vi "test_CCDSetAndGetGain.vi"(6 "Delay between send and receive [ms]":i32=100, 7 "Test should pass":bool=TRUE, 8 "error in":errorcluster, 9 "tear down connection":bool=TRUE, 10 "set-up a connection":bool=TRUE, 11 "device selection":enum16{"monochromator", "CCD", "SCD"}(ring)=enum."CCD") -> (0 "error out":errorcluster)   [LabVIEW 2023]
uses:
  Classes/CCD/GainTokenEnum.ctl
  Classes/CCD/CCD.lvclass
  <vilib>/addons/_JKI Toolkits/Caraya/classes/Assert/Assert Equal Value and Type_Variant.vi
  <vilib>/addons/_JKI Toolkits/Caraya/classes/Assert/Assert Not Error.vi
  <vilib>/addons/_JKI Toolkits/Caraya/classes/Test/Test.lvclass
  <vilib>/addons/_JKI Toolkits/Caraya/classes/Assert/Assert.lvclass
panel:
  # "Connector Pane"
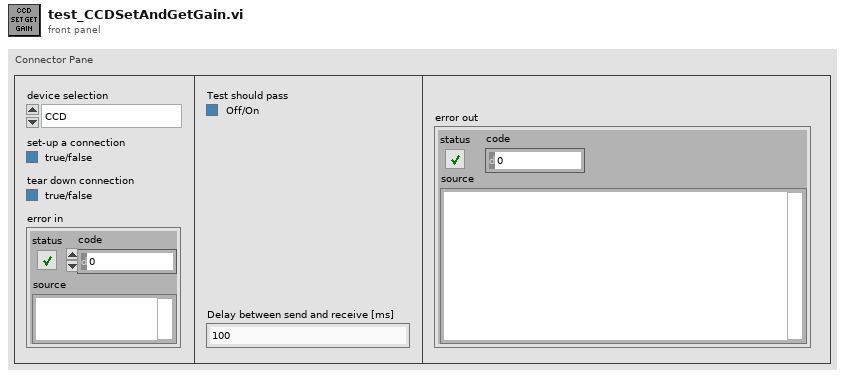
[diagram p1: front panel]
types:
  T1 = typedef "CCD.lvclass/GainTokenEnum.ctl" = enum16{"High Light", "Best Dynamic Range", "High Sensitivity"}
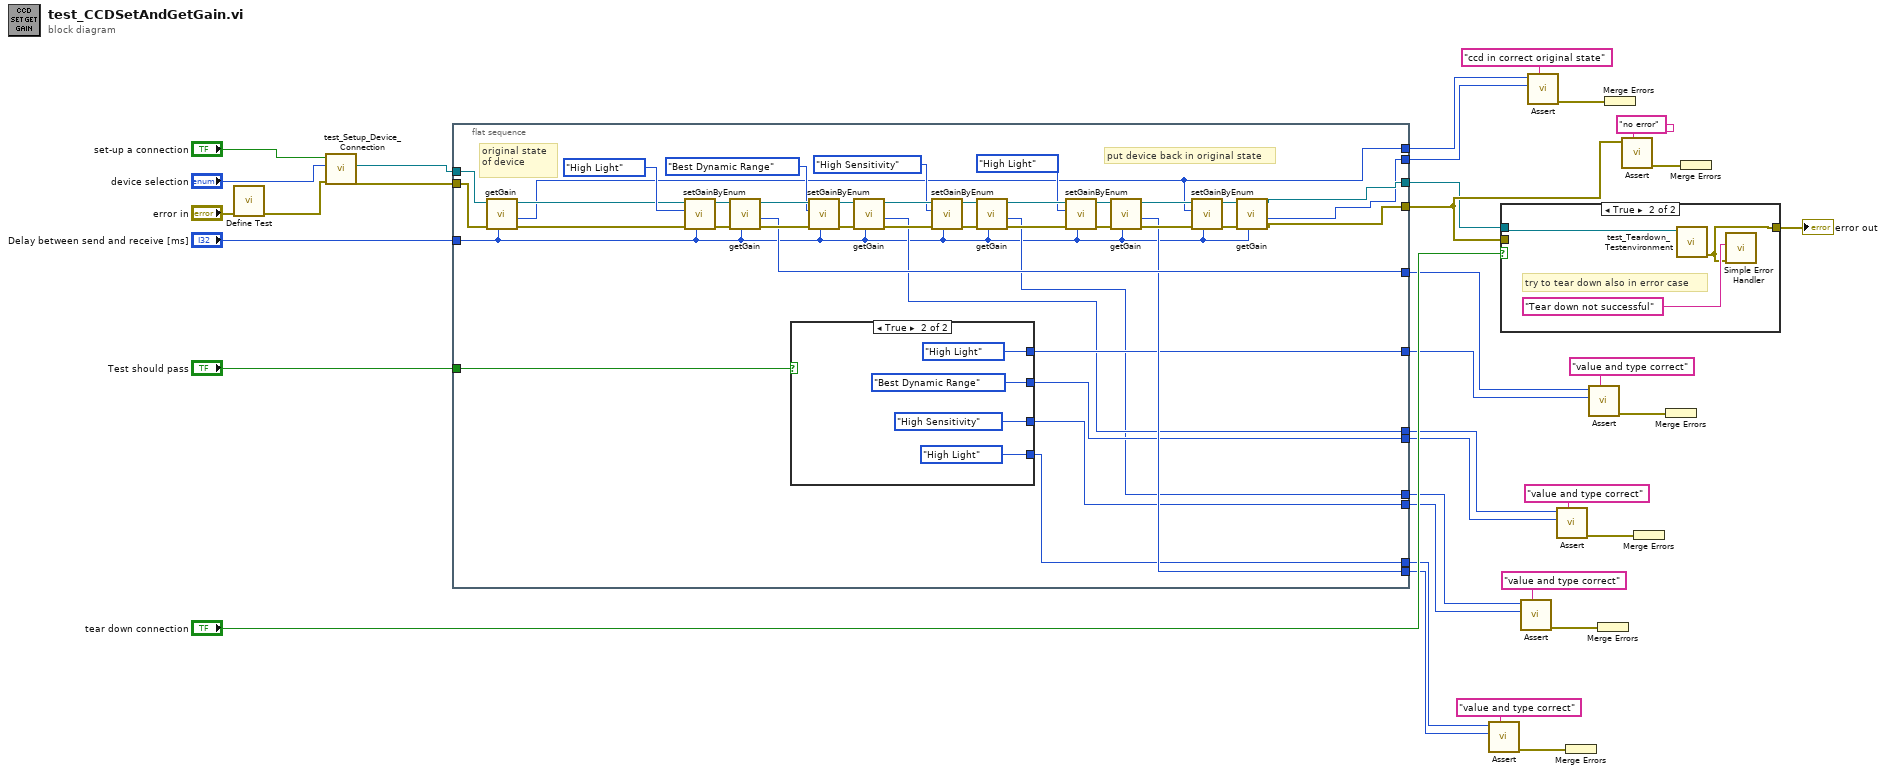
[diagram p0: block diagram]
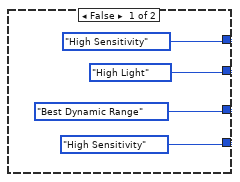
[diagram p2: hidden frame]
diagram:
  n1 = call <vilib>:"Define Test.vi"("error in (no error)"="error in") -> ("error out"=w4:errorcluster)  [unwired: 9 in, 1 out]
  n2 = call "test_Setup_Device_Connection.vi"("error in (no error)"=w4, "device selection"="device selection", "set-up a connection"="set-up a connection") -> ("error out"=w5:errorcluster, "CCD.lvclass"=w6:refnum<class "CCD.lvclass">)  [unwired: 5 in, 2 out]
  n3 = flat-sequence {
    tunnel: w5 -> [w72]
    tunnel: w6 -> [w73]
    tunnel: [w46] -> w27
    tunnel: "Test should pass" -> [w74]
    tunnel: [w45] -> w26
    tunnel: [w44] -> w23
    tunnel: [w47] -> w22
    tunnel: [w43] -> w21
    tunnel: [w40] -> w19
    tunnel: [w36] -> w17
    tunnel: [w42] -> w14
    tunnel: [w41] -> w20
    tunnel: [w39] -> w18
    tunnel: [w37] -> w16
    tunnel: [w38] -> w15
    tunnel: "Delay between send and receive [ms]" -> [w35]
    frame #0 {
      # "put device back in original state"
      # "original state of device"
      n4 = call "getGain.vi"("Delay between send and receive [ms]"=w35, "error in (no error)"=w72, "CCD in"=w73) -> ("error out"=w48:errorcluster, "gain token (enum)"=w47:T1, "CCD out"=w49:refnum<class "CCD.lvclass">)  [unwired: 5 in, 1 out]
      n5 = call "setGainByEnum.vi"("Delay between send and receive [ms]"=w35, "error in (no error)"=w48, "gain"=GainTokenEnum."High Light" ("gain token (enum)"), "CCD in"=w49) -> ("error out"=w61:errorcluster, "CCD out"=w60:refnum<class "CCD.lvclass">)  [unwired: 4 in, 2 out]
      n6 = call "getGain.vi"("Delay between send and receive [ms]"=w35, "error in (no error)"=w61, "CCD in"=w60) -> ("error out"=w65:errorcluster, "gain token (enum)"=w43:T1, "CCD out"=w64:refnum<class "CCD.lvclass">)  [unwired: 5 in, 1 out]
      n7 = case shown="True" w74 {
        tunnel: [GainTokenEnum."High Sensitivity" ("gain token (enum)") GainTokenEnum."High Light" ("gain token (enum)")] -> w41
        tunnel: [GainTokenEnum."High Light" ("gain token (enum)") GainTokenEnum."Best Dynamic Range" ("gain token (enum)")] -> w39
        tunnel: [GainTokenEnum."Best Dynamic Range" ("gain token (enum)") GainTokenEnum."High Sensitivity" ("gain token (enum)")] -> w37
        tunnel: [GainTokenEnum."High Sensitivity" ("gain token (enum)") GainTokenEnum."High Light" ("gain token (enum)")] -> w38
        frame False {
        }
        frame True {
        }
      }
      n8 = call "setGainByEnum.vi"("Delay between send and receive [ms]"=w35, "error in (no error)"=w65, "gain"=GainTokenEnum."Best Dynamic Range" ("gain token (enum)"), "CCD in"=w64) -> ("error out"=w62:errorcluster, "CCD out"=w63:refnum<class "CCD.lvclass">)  [unwired: 4 in, 2 out]
      n9 = call "getGain.vi"("Delay between send and receive [ms]"=w35, "error in (no error)"=w62, "CCD in"=w63) -> ("error out"=w67:errorcluster, "gain token (enum)"=w40:T1, "CCD out"=w66:refnum<class "CCD.lvclass">)  [unwired: 5 in, 1 out]
      n10 = call "setGainByEnum.vi"("Delay between send and receive [ms]"=w35, "error in (no error)"=w67, "gain"=GainTokenEnum."High Sensitivity" ("gain token (enum)"), "CCD in"=w66) -> ("error out"=w55:errorcluster, "CCD out"=w54:refnum<class "CCD.lvclass">)  [unwired: 4 in, 2 out]
      n11 = call "getGain.vi"("Delay between send and receive [ms]"=w35, "error in (no error)"=w55, "CCD in"=w54) -> ("error out"=w59:errorcluster, "gain token (enum)"=w36:T1, "CCD out"=w58:refnum<class "CCD.lvclass">)  [unwired: 5 in, 1 out]
      n12 = call "setGainByEnum.vi"("Delay between send and receive [ms]"=w35, "error in (no error)"=w59, "gain"=GainTokenEnum."High Light" ("gain token (enum)"), "CCD in"=w58) -> ("error out"=w56:errorcluster, "CCD out"=w57:refnum<class "CCD.lvclass">)  [unwired: 4 in, 2 out]
      n13 = call "getGain.vi"("Delay between send and receive [ms]"=w35, "error in (no error)"=w56, "CCD in"=w57) -> ("error out"=w71:errorcluster, "gain token (enum)"=w42:T1, "CCD out"=w70:refnum<class "CCD.lvclass">)  [unwired: 5 in, 1 out]
      n14 = call "setGainByEnum.vi"("Delay between send and receive [ms]"=w35, "error in (no error)"=w71, "gain"=w47, "CCD in"=w70) -> ("error out"=w68:errorcluster, "CCD out"=w69:refnum<class "CCD.lvclass">)  [unwired: 4 in, 2 out]
      n15 = call "getGain.vi"("Delay between send and receive [ms]"=w35, "error in (no error)"=w68, "CCD in"=w69) -> ("error out"=w46:errorcluster, "gain token (enum)"=w44:T1, "CCD out"=w45:refnum<class "CCD.lvclass">)  [unwired: 5 in, 1 out]
    }
  }
  n16 = call-poly <vilib>:"Assert.vi"("Label"="value and type correct" ("Label (VI Title)"), "Y"=w14, "X"=w15) -> ("error out"=w33:errorcluster)  [unwired: 7 in, 1 out]
  n17 = case shown="True" "tear down connection" {
    tunnel: w26 -> [_ w85]
    tunnel: [w83 w84] -> w7
    tunnel: w27 -> [w83 _]
    frame False {
    }
    frame True {
      # "try to tear down also in error case"
      n18 = call "test_Teardown_Testenvironment.vi"("GenericDevice.lvclass"=w85) -> ("error out"=w84:errorcluster)  [unwired: 9 in, 1 out]
      n19 = call <vilib>:"Simple Error Handler.vi"("error source (\" \")"="Tear down not successful" ("error source (\" \")"), "error in (no error)"=w84) -> ()  [unwired: 3 in, 5 out]
    }
  }
  "error out" <- w7
  n20 = call-poly <vilib>:"Assert.vi"("Label"="value and type correct" ("Label (VI Title)"), "Y"=w16, "X"=w17) -> ("error out"=w13:errorcluster)  [unwired: 7 in, 1 out]
  n21 = call-poly <vilib>:"Assert.vi"("Label"="ccd in correct original state" ("Label (VI Title)"), "Y"=w23, "X"=w22) -> ("error out"=w25:errorcluster)  [unwired: 7 in, 1 out]
  n22 = call-poly <vilib>:"Assert.vi"("Label"="value and type correct" ("Label (VI Title)"), "Y"=w18, "X"=w19) -> ("error out"=w9:errorcluster)  [unwired: 7 in, 1 out]
  n23 = Merge Errors(w33) -> ()  [unwired: 1 out]
  n24 = call-poly <vilib>:"Assert.vi"("Label"="value and type correct" ("Label (VI Title)"), "Y"=w20, "X"=w21) -> ("error out"=w10:errorcluster)  [unwired: 7 in, 1 out]
  n25 = Merge Errors(w13) -> ()  [unwired: 1 out]
  n26 = Merge Errors(w25) -> ()  [unwired: 1 out]
  n27 = call-poly <vilib>:"Assert.vi"("Label"="no error" ("Label (VI Title)"), "Not Error?"=w27) -> ("error out"=w29:errorcluster)  [unwired: 8 in, 1 out]
  n28 = Merge Errors(w9) -> ()  [unwired: 1 out]
  n29 = Merge Errors(w10) -> ()  [unwired: 1 out]
  n30 = Merge Errors(w29) -> ()  [unwired: 1 out]
